vi "Init Msg Output.vi"() -> (3 "Start Msg Output out":refnum<class "Start Msg Output.lvclass">)   [LabVIEW 2020, in "jettl.lvlib" / "Start jettl Msg.lvlib" / "Start Msg Output.lvlib" / "Start Msg Output.lvclass"]
doc: "jettl 6.14.1.98\nNathan Davis - Nathan Davis\nCopyright (c) 2026, Nathan Davis\nMIT"
uses:
  Start Msg Output.lvclass
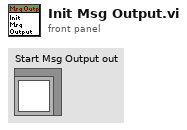
[diagram p1: front panel]
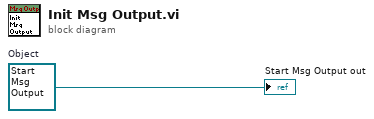
[diagram p0: block diagram]
diagram:
  w1 = refnum<class "Start Msg Output.lvclass"> refnum  # Object
  "Start Msg Output out" <- w1
